vi "Gyro Angle.vi"() -> (1 "Rate":dbl, 3 "Angle":dbl)   [LabVIEW 2013]
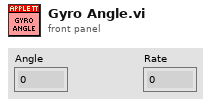
[diagram p1: front panel]
types:
  T1 = typedef "WPI_GyroDevRef.ctl" = cluster{"DevStatus":errorcluster, "Analog Module":T2, "Analog Channel":T3, "Offset":dbl, "Gain (VoltsPerDegree/Second)":dbl}
  T2 = typedef "FPGA_TypedefAnalogModule.ctl" = enum16{"Analog Module 1", "Analog Module 2"}
  T3 = typedef "FPGA_AIChannel.ctl" = enum8{"AI 1", "AI 2", "AI 3", "AI 4", "AI 5", "AI 6", "AI 7", "AI 8", "Invalid"}
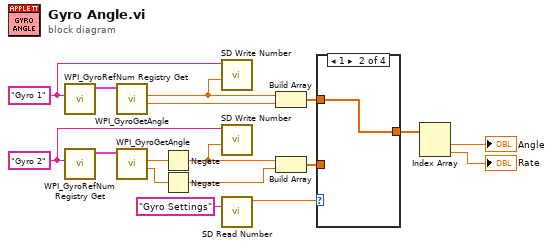
[diagram p0: block diagram]
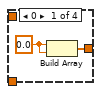
[diagram p2: hidden frame]
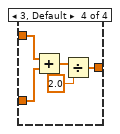
[diagram p4: hidden frame]
diagram:
  w13 = "Gyro 2" ("refnum name")
  w12 = "Gyro 1" ("refnum name")
  n1 = call <vilib>:"WPI_GyroRefNum Registry Get.vi"("refnum name"=w12) -> ("GyroDevRef"=w11:T1)  [unwired: 9 in, 1 out]
  n2 = call <vilib>:"WPI_GyroRefNum Registry Get.vi"("refnum name"=w13) -> ("GyroDevRef"=w14:T1)  [unwired: 9 in, 1 out]
  n3 = call <vilib>:"WPI_GyroGetAngle.vi"("GyroDevRef"=w11) -> ("Angular Rate"=w10:dbl, "Angle"=w9:dbl)  [unwired: 7 in, 2 out]
  n4 = call <vilib>:"WPI_GyroGetAngle.vi"("GyroDevRef"=w14) -> ("Angular Rate"=w6:dbl, "Angle"=w17:dbl)  [unwired: 7 in, 2 out]
  n5 = Negate(x=w17) -> (-x=w7:dbl)
  n6 = Negate(x=w6) -> (-x=w5:dbl)
  n7 = call <vilib>:"SD Write Number.vi"("Numeric"=w9, "Name"=w12) -> ()  [unwired: 8 in, 2 out]
  n8 = call <vilib>:"SD Write Number.vi"("Numeric"=w7, "Name"=w13) -> ()  [unwired: 8 in, 2 out]
  n9 = call <vilib>:"SD Read Number.vi"("Name"="Gyro Settings") -> ("Numeric"=w16:dbl)  [unwired: 8 in, 2 out]
  n10 = Build Array(w9, w10) -> (w8:dbl[])
  n11 = Build Array(w7, w5) -> (w4:dbl[])
  n12 = case shown="1" w16 {
    tunnel: w8 -> [_ w20 _ w23]
    tunnel: w4 -> [_ _ w21 w24]
    tunnel: [w19 w20 w21 w22] -> w3
    frame 0 {
      w18 = 0.0 ("x")
      n13 = Build Array(w18, w18) -> (w19:dbl[])
    }
    frame 1 {
    }
    frame 2 {
    }
    frame 3, Default {
      n14 = Add(x=w23, y=w24) -> (x+y=w26:dbl[])
      n15 = Divide(x=w26, y=2.0) -> (x/y=w22:dbl[])
    }
  }
  n16 = Index Array(array=w3) -> (element #1=→"Angle":dbl, element #2=→"Rate":dbl)  [unwired: 2 in]
